vi "Continuous_Measurement_v4.vi"() -> ()   [LabVIEW 2014]
uses:
  <vilib>/Analysis/NI_AALBase.lvlib
panel:
  out "Redraw V-I graph?":bool
  in  "Reset Graphs?":bool
  out "File Startname":string
  in  "stop":bool
  out "I-t Graph":dbl[](graph)
  out "V-t Graph":dbl[](graph)
  out "V-I Graph":cluster{dbl[], dbl[]}(graph)
  in  "Meas. wait time (ms)":i32
  in  "Meas. to Avg":i32
  out "Voltage (V)":string
  in  "Current (uA)":dbl
  in  "Collect":bool
  in  "Outp. wait time (ms)":i32
  in  "2182A VISA":refnum<visa-resource-name>
  in  "Output Response":bool
  in  "Compliance (V)":dbl
  out "File Counter":i32
  out "Data Counter":i32
  in  "6221 VISA":refnum<visa-resource-name>
  in  "First Path":path
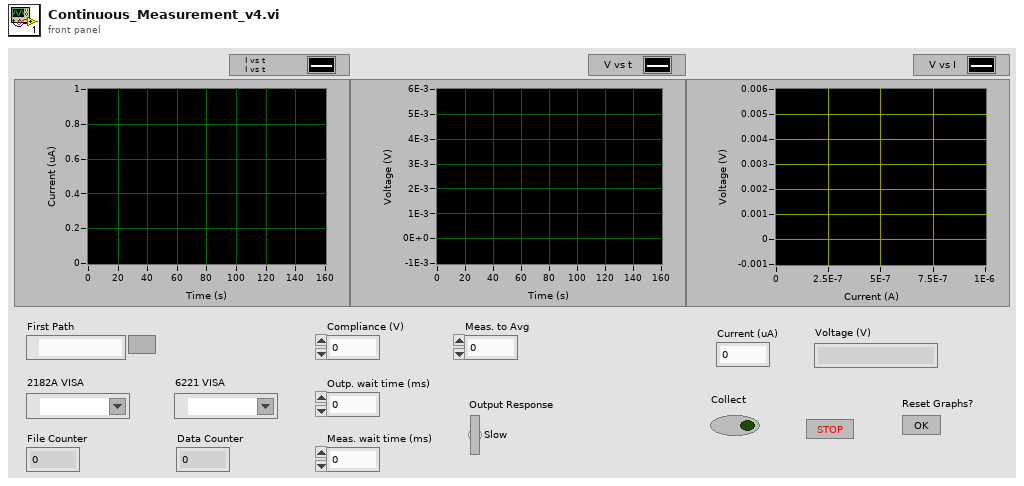
[diagram p1: front panel]
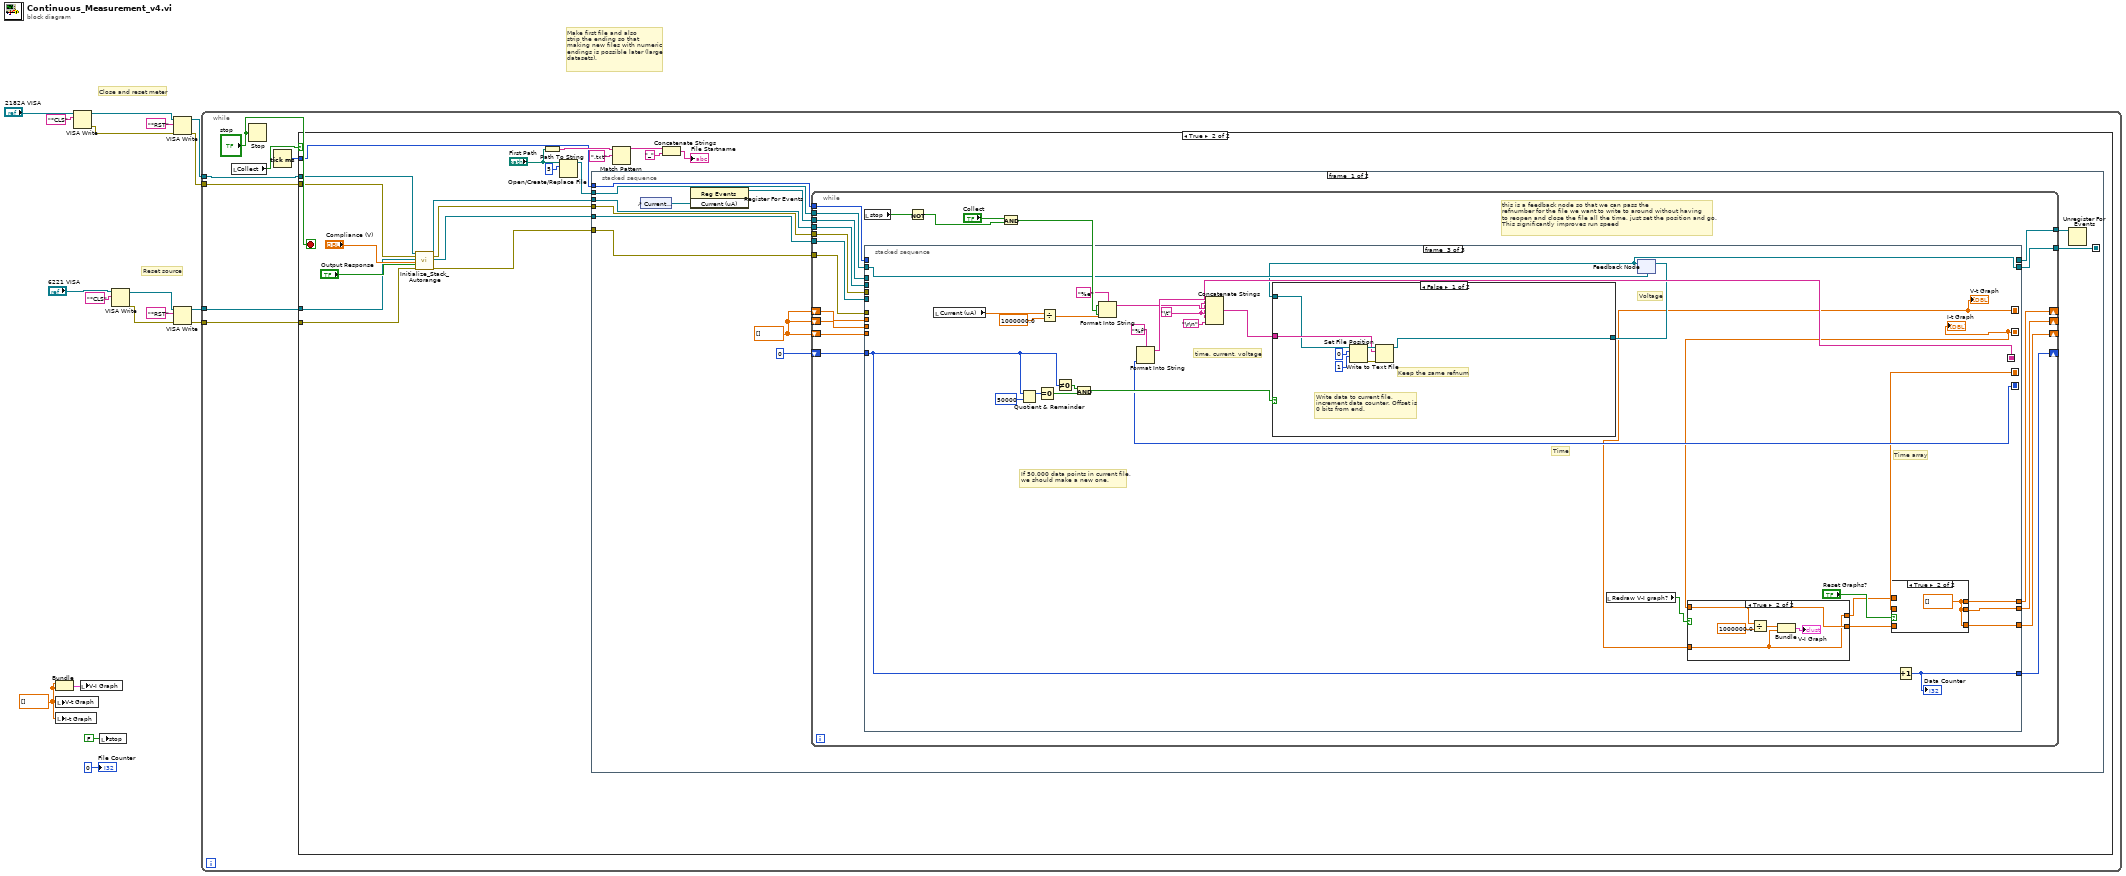
[diagram p0: block diagram]
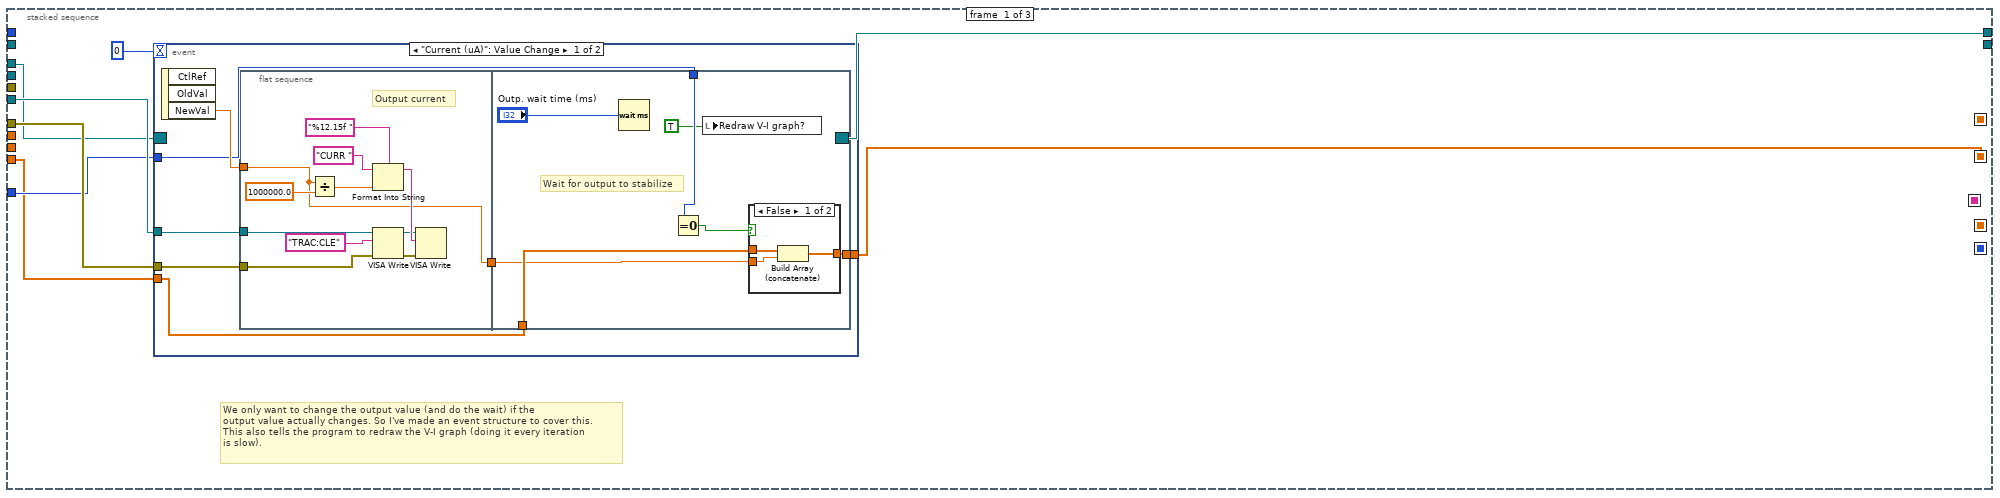
[diagram p3: hidden frame]
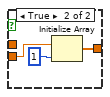
[diagram p4: hidden frame]
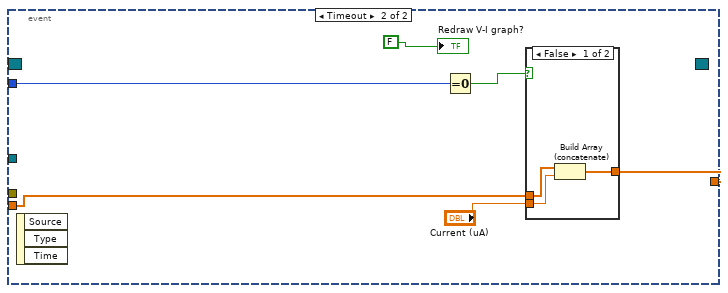
[diagram p5: hidden frame]
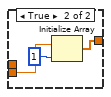
[diagram p6: hidden frame]
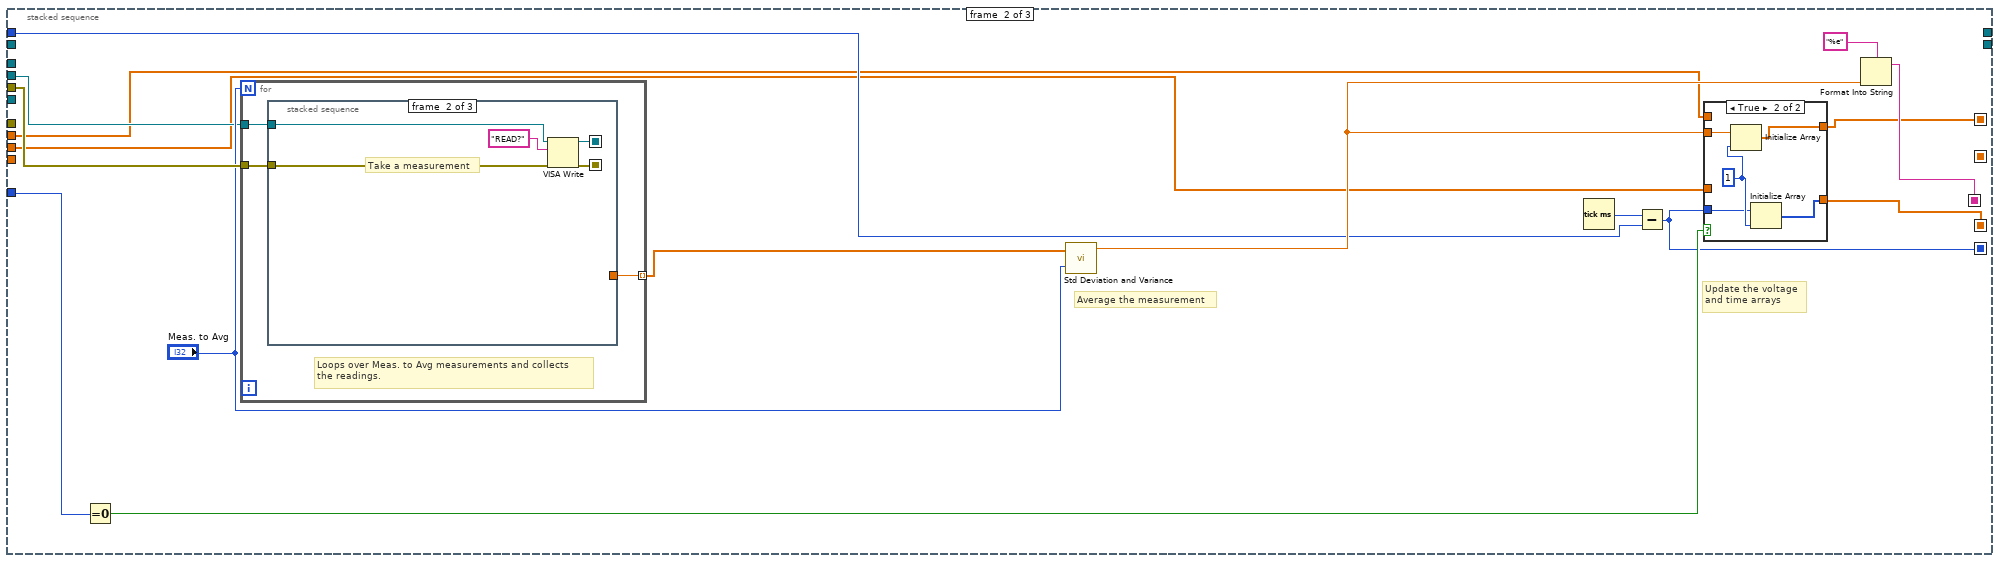
[diagram p7: hidden frame]
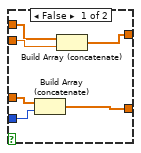
[diagram p8: hidden frame]
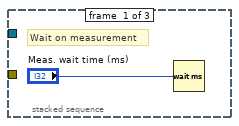
[diagram p9: hidden frame]
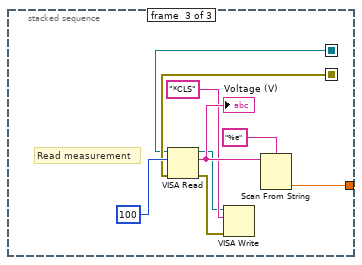
[diagram p10: hidden frame]
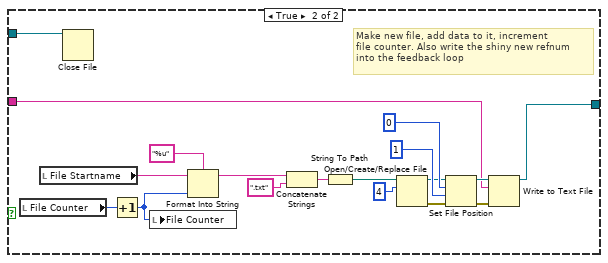
[diagram p13: hidden frame]
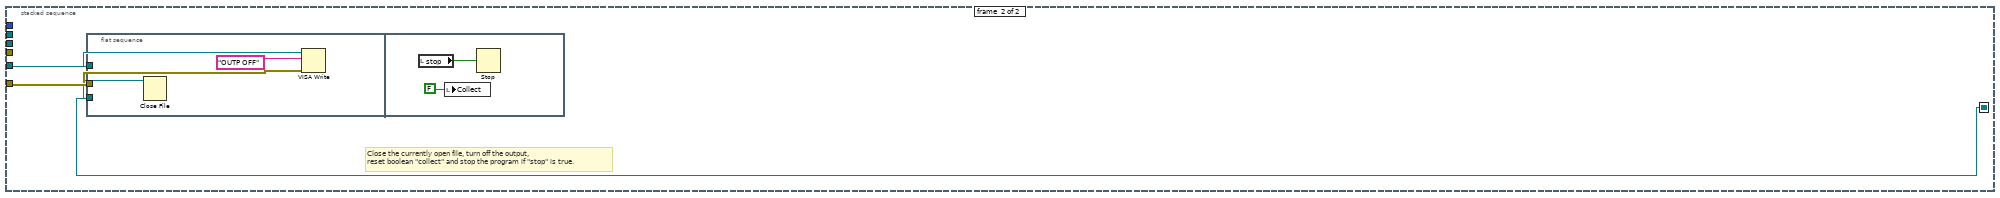
[diagram p14: hidden frame]
diagram:
  w2 = dbl[] []
  # "Make first file and also\nstrip the ending so that\nmaking new files with numeric\nendings is possible later (large\ndatasets)."
  # "Reset source"
  # "Close and reset meter"
  n1 = Bundle(w2, w2) -> (w1:cluster{dbl[], dbl[]})  [unwired: 1 in]
  n2 = local write "V-t Graph"(w2) -> ()
  n3 = local write "I-t Graph"(w2) -> ()
  n4 = VISA Write(VISA resource name="2182A VISA", write buffer="*CLS") -> (VISA resource name out=w11:refnum<visa-resource-name>, error out=w15:errorcluster)  [unwired: 1 in, 1 out]
  n5 = local write "V-I Graph"(w1) -> ()
  n6 = local write "stop"(FALSE) -> ()
  n7 = VISA Write(VISA resource name="6221 VISA", write buffer="*CLS") -> (VISA resource name out=w4:refnum<visa-resource-name>, error out=w5:errorcluster)  [unwired: 1 in, 1 out]
  n8 = VISA Write(VISA resource name=w11, write buffer="*RST", error in (no error)=w15) -> (VISA resource name out=w10:refnum<visa-resource-name>, error out=w9:errorcluster)  [unwired: 1 out]
  n9 = VISA Write(VISA resource name=w4, write buffer="*RST", error in (no error)=w5) -> (VISA resource name out=w7:refnum<visa-resource-name>, error out=w6:errorcluster)  [unwired: 1 out]
  n10 = while {
    tunnel: w10 -> [w24]
    tunnel: w9 -> [w23]
    tunnel: w7 -> [w22]
    tunnel: w6 -> [w21]
    stop <- "stop" stop-if-true
    n11 = local read "Collect"() -> (w25:bool)
    n12 = Stop(stop? (T)="stop") -> ()
    n13 = Tick Count (ms)() -> (millisecond timer value=w19:u32)
    n14 = case shown="True" w25 {
      tunnel: w23 -> [_ w30]
      tunnel: w24 -> [_ w31]
      tunnel: w22 -> [_ w32]
      tunnel: w21 -> [_ w33]
      tunnel: w19 -> [_ w36]
      frame False {
      }
      frame True {
        n15 = call "Initialize_Stack_Autorange.vi"("2182A VISA in"=w31, "21282A Error In"=w30, "6221 VISA in"=w32, "Compliance (V)"="Compliance (V)", "Output Response"="Output Response", "6221 Error In"=w33) -> ("2182A VISA out"=w29:refnum<visa-resource-name>, "2182A Error Out"=w28:errorcluster, "6221 VISA out"=w27:refnum<visa-resource-name>, "6221 Error Out"=w26:errorcluster)  [unwired: 10 in]
        n16 = Path To String(path="First Path") -> (string=w43:string)
        n17 = Open/Create/Replace File(file path (use dialog)="First Path", operation (0:open)=5) -> (refnum out=w40:refnum<file>)  [unwired: 4 in, 2 out]
        n18 = stacked-sequence {
          seq-local: [w51 _] -> [_ w242]
          tunnel: w26 -> [w56 w243]
          tunnel: w28 -> [w55 _]
          tunnel: w27 -> [w54 w244]
          tunnel: w29 -> [w53 _]
          tunnel: w40 -> [w52 _]
          tunnel: w36 -> [w48 _]
          frame #0 {
            w47 = dbl[] []
            n19 = control-ref of="Current (uA)"() -> (w50:refnum<vi>)
            n20 = register-events(w50) -> (reference out=w49:refnum<event-registration>)  [unwired: 2 in, 1 out]
            n21 = while {
              tunnel: w56 -> [w77]
              tunnel: w55 -> [w68]
              tunnel: w54 -> [w73]
              tunnel: w53 -> [w67]
              tunnel: w52 -> [w71]
              tunnel: [w70] -> w51
              tunnel: w49 -> [w69]
              tunnel: w48 -> [w66]
              shift-right: [w59] -> _
              shift-left: w47 -> [w60]
              shift-right: [w58] -> _
              shift-left: w47 -> [w62]
              shift-right: [w57] -> _
              shift-left: w47 -> [w65]
              shift-right: [w64] -> _
              shift-left: 0 -> [w63]
              tunnel: [w61] -> w45
              stop <- w74 continue-if-true
              # "this is a feedback node so that we can pass the\nrefnumber for the file we want to write to around without having\nto reopen and close the file all the time, just set the position and go. \nThis significantly improves run speed"
              n22 = local read "stop"() -> (w72:bool)
              n23 = stacked-sequence {
                seq-local: [_ w140 _] -> [_ _ w196]
                seq-local: [w80 _ _] -> [_ _ w176]
                seq-local: [_ w132 _] -> [_ _ w178]
                seq-local: [_ w131 _] -> [_ _ w183]
                seq-local: [_ w130 _] -> [_ _ w182]
                tunnel: w77 -> [w84 _ _]
                tunnel: w68 -> [_ w144 _]
                tunnel: w73 -> [w85 _ _]
                tunnel: w67 -> [_ w139 _]
                tunnel: w71 -> [_ _ w192]
                tunnel: [_ _ w190] -> w70
                tunnel: w69 -> [w83 _ _]
                tunnel: w66 -> [_ w136 _]
                tunnel: w65 -> [_ w133 _]
                tunnel: [_ _ w185] -> w64
                tunnel: w63 -> [w81 w135 w186]
                tunnel: w62 -> [w79 _ _]
                tunnel: [w78 _ _] -> w61
                tunnel: w60 -> [_ w129 _]
                tunnel: [_ _ w181] -> w59
                tunnel: [_ _ w180] -> w58
                tunnel: [_ _ w179] -> w57
                frame #0 {
                  # "We only want to change the output value (and do the wait) if the\noutput value actually changes. So I've made an event structure to cover this.\nThis also tells the program to redraw the V-I graph (doing it every iteration\nis slow)."
                  n24 = event shown="[0] \"Current (uA)\": Value Change" {
                    selector: w83 -> [_ _]
                    dyn-events: [_ _] -> w78
                    timeout: 0 -> [_ _]
                    tunnel: w85 -> [w91 _]
                    tunnel: w84 -> [w90 _]
                    tunnel: w81 -> [w89 w120]
                    tunnel: [w88 w119] -> w80
                    tunnel: w79 -> [w86 w118]
                    event "Current (uA)": Value Change {
                      n25 = event-data() -> ("NewVal"=w92:dbl)  [unwired: 1 in, 2 out]
                      n26 = flat-sequence {
                        tunnel: w92 -> [w93]
                        tunnel: w91 -> [w95]
                        tunnel: w90 -> [w94]
                        tunnel: [w93] -> w87
                        tunnel: w86 -> [w106]
                        tunnel: w89 -> [w109]
                        tunnel: [w107] -> w88
                        tunnel: w87 -> [w105]
                        frame #0 {
                          # "Output current"
                          n27 = Divide(x=w93, y=1000000.0) -> (x/y=w98:dbl)
                          n28 = Format Into String(format string="%12.15f ", initial string="CURR ", w98) -> (resulting string=w100:string)  [unwired: 1 in, 1 out]
                          n29 = VISA Write(VISA resource name=w95, write buffer="TRAC:CLE", error in (no error)=w94) -> (VISA resource name out=w97:refnum<visa-resource-name>, error out=w102:errorcluster)  [unwired: 1 out]
                          n30 = VISA Write(VISA resource name=w97, write buffer=w100, error in (no error)=w102) -> ()  [unwired: 3 out]
                        }
                        frame #1 {
                          # "Wait for output to stabilize"
                          n31 = Wait (ms)(milliseconds to wait="Outp. wait time (ms)") -> ()  [unwired: 1 out]
                          n32 = Equal To 0?(x=w109) -> (x = 0?=w108:bool)
                          n33 = local write "Redraw V-I graph?"(TRUE) -> ()
                          n34 = case shown="False" w108 {
                            tunnel: [w111 w115] -> w107
                            tunnel: w105 -> [w112 w114]
                            tunnel: w106 -> [w113 _]
                            frame False {
                              n35 = Build Array (concatenate)(w113, w112) -> (w111:dbl[])
                            }
                            frame True {
                              n36 = Initialize Array(w114, 1) -> (w115:dbl[])
                            }
                          }
                        }
                      }
                    }
                    event Timeout {
                      n37 = event-data() -> ()  [unwired: 1 in, 3 out]
                      n38 = Equal To 0?(x=w120) -> (x = 0?=w121:bool)
                      n39 = case shown="False" w121 {
                        tunnel: [w123 w127] -> w119
                        tunnel: "Current (uA)" -> [w124 w126]
                        tunnel: w118 -> [w125 _]
                        frame False {
                          n40 = Build Array (concatenate)(w125, w124) -> (w123:dbl[])
                        }
                        frame True {
                          n41 = Initialize Array(w126, 1) -> (w127:dbl[])
                        }
                      }
                      "Redraw V-I graph?" <- FALSE
                    }
                  }
                }
                frame #1 {
                  # "Update the voltage\nand time arrays"
                  # "Average the measurement"
                  n42 = Equal To 0?(x=w135) -> (x = 0?=w134:bool)
                  n43 = for {
                    N: "Meas. to Avg" -> [_]
                    tunnel: w144 -> [w158]
                    tunnel: [w157] -> w143 mode=indexing
                    tunnel: w139 -> [w156]
                    # "Loops over Meas. to Avg measurements and collects\nthe readings."
                    n44 = stacked-sequence {
                      seq-local: [_ w162 _] -> [_ _ w172]
                      seq-local: [_ w160 _] -> [_ _ w169]
                      tunnel: w158 -> [_ w163 _]
                      tunnel: [_ _ w170] -> w157
                      tunnel: w156 -> [_ w161 _]
                      frame #0 {
                        # "Wait on measurement"
                        n45 = Wait (ms)(milliseconds to wait="Meas. wait time (ms)") -> ()  [unwired: 1 out]
                      }
                      frame #1 {
                        # "Take a measurement"
                        n46 = VISA Write(VISA resource name=w161, write buffer="READ?", error in (no error)=w163) -> (VISA resource name out=w160:refnum<visa-resource-name>, error out=w162:errorcluster)  [unwired: 1 out]
                      }
                      frame #2 {
                        # "Read measurement"
                        n47 = VISA Read(VISA resource name=w169, byte count=100, error in (no error)=w172) -> (VISA resource name out=w166:refnum<visa-resource-name>, read buffer=w168:string, error out=w165:errorcluster)  [unwired: 1 out]
                        "Voltage (V)" <- w168
                        n48 = VISA Write(VISA resource name=w166, write buffer="*CLS", error in (no error)=w165) -> ()  [unwired: 3 out]
                        n49 = Scan From String(format string="%e", input string=w168) -> (output 1=w170:dbl)  [unwired: 3 in, 3 out]
                      }
                    }
                  }
                  n50 = call <vilib>:"Std Deviation and Variance.vi"("X"=w143, "Weighting (Sample)"="Meas. to Avg") -> ("mean"=w138:dbl)  [unwired: 2 out]
                  n51 = Tick Count (ms)() -> (millisecond timer value=w137:u32)
                  n52 = Subtract(x=w137, y=w136) -> (x-y=w131:u32)
                  n53 = case shown="True" w134 {
                    tunnel: w131 -> [w150 w154]
                    tunnel: w138 -> [w149 w153]
                    tunnel: [w148 w152] -> w132
                    tunnel: [w147 w151] -> w130
                    tunnel: w129 -> [w146 _]
                    tunnel: w133 -> [w145 _]
                    frame False {
                      n54 = Build Array (concatenate)(w145, w150) -> (w148:dbl[])
                      n55 = Build Array (concatenate)(w146, w149) -> (w147:dbl[])
                    }
                    frame True {
                      w155 = 1
                      n56 = Initialize Array(w153, w155) -> (w151:dbl[])
                      n57 = Initialize Array(w154, w155) -> (w152:u32[])
                    }
                  }
                  n58 = Format Into String(format string="%e", w138) -> (resulting string=w140:string)  [unwired: 2 in, 1 out]
                }
                frame #2 {
                  w201 = "\t"
                  # "Voltage"
                  # "Time array"
                  # "Time"
                  # "time, current, voltage"
                  # "If 50,000 data points in current file,\nwe should make a new one."
                  n59 = local read "Current (uA)"() -> (w184:dbl)
                  n60 = Quotient & Remainder(x=w186, y=50000) -> (x-y*floor(x/y)=w193:i32)  [unwired: 1 out]
                  n61 = Equal To 0?(x=w193) -> (x = 0?=w188:bool)
                  n62 = Divide(x=w184, y=1000000.0) -> (x/y=w195:dbl)
                  n63 = Not Equal To 0?(x=w186) -> (x != 0?=w187:bool)
                  n64 = And(x=w187, y=w188) -> (x .and. y?=w198:bool)
                  n65 = Format Into String(format string="%e", w195) -> (resulting string=w202:string)  [unwired: 2 in, 1 out]
                  n66 = Format Into String(format string="%f", w183) -> (resulting string=w204:string)  [unwired: 2 in, 1 out]
                  n67 = Concatenate Strings(w204, w201, w202, w201, w196, "\r\n") -> (w197:string)
                  n68 = local read "Redraw V-I graph?"() -> (w177:bool)
                  n69 = feedback #1(w192) -> (w190:refnum<file>)
                  n70 = case shown="False" w198 {
                    tunnel: w197 -> [w220 w231]
                    tunnel: [w218 w230] -> w191
                    tunnel: w190 -> [w217 w241]
                    frame False {
                      # "Keep the same refnum"
                      # "Write data to current file,\nincrement data counter. Offset is\n0 bits from end."
                      n71 = Set File Position(offset (in bytes) (0)=0, refnum=w217, from (0:start)=1) -> (refnum out=w221:refnum<file>, error out=w219:errorcluster)  [unwired: 1 in]
                      n72 = Write to Text File(file (use dialog)=w221, text=w220, error in=w219) -> (refnum out=w218:refnum<file>)  [unwired: 1 in, 2 out]
                    }
                    frame True {
                      # "Make new file, add data to it, increment\nfile counter. Also write the shiny new refnum\ninto the feedback loop"
                      n73 = local read "File Counter"() -> (w229:i32)
                      n74 = local read "File Startname"() -> (w224:string)
                      n75 = Close File(refnum=w241) -> ()  [unwired: 1 in, 2 out]
                      n76 = Increment(x=w229) -> (x+1=w225:i32)
                      n77 = local write "File Counter"(w225) -> ()
                      n78 = Format Into String(format string="%u", initial string=w224, w225) -> (resulting string=w240:string)  [unwired: 1 in, 1 out]
                      n79 = Concatenate Strings(w240, ".txt") -> (w236:string)
                      n80 = String To Path(string=w236) -> (path=w238:path)
                      n81 = Open/Create/Replace File(file path (use dialog)=w238, operation (0:open)=u16 4) -> (refnum out=w228:refnum<file>, error out=w227:errorcluster)  [unwired: 4 in, 1 out]
                      n82 = Set File Position(offset (in bytes) (0)=i64 0, refnum=w228, from (0:start)=u16 1, error in=w227) -> (refnum out=w234:refnum<file>, error out=w235:errorcluster)
                      n83 = Write to Text File(file (use dialog)=w234, text=w231, error in=w235) -> (refnum out=w230:refnum<file>)  [unwired: 1 in, 2 out]
                    }
                  }
                  n84 = feedback-in #1(w191) -> ()
                  n85 = case shown="True" w177 {
                    tunnel: w176 -> [w207 w209]
                    tunnel: w182 -> [w206 w208]
                    tunnel: [w207 w209] -> w175
                    tunnel: [w206 w208] -> w174
                    frame False {
                    }
                    frame True {
                      n86 = Divide(x=w209, y=1000000.0) -> (x/y=w211:dbl[])
                      n87 = Bundle(w211, w208) -> (→"V-I Graph":cluster{dbl[], dbl[]})  [unwired: 1 in]
                    }
                  }
                  n88 = case shown="True" "Reset Graphs?" {
                    tunnel: [w214 w216] -> w181
                    tunnel: [w215 w216] -> w180
                    tunnel: w175 -> [w215 _]
                    tunnel: w174 -> [w214 _]
                    tunnel: [w213 w216] -> w179
                    tunnel: w178 -> [w213 _]
                    frame False {
                    }
                    frame True {
                      w216 = dbl[] []
                    }
                  }
                  n89 = Increment(x=w186) -> (x+1=w185:i32)
                  "Data Counter" <- w185
                  "V-t Graph" <- w182
                  "I-t Graph" <- w176
                }
              }
              n90 = Not(x=w72) -> (.not. x?=w75:bool)
              n91 = And(x="Collect", y=w75) -> (x .and. y?=w74:bool)
            }
            n92 = Unregister For Events(event registration refnum=w45) -> ()  [unwired: 1 in, 1 out]
          }
          frame #1 {
            # "Close the currently open file, turn off the output,\nreset boolean \"collect\" and stop the program if \"stop\" is true."
            n93 = flat-sequence {
              tunnel: w244 -> [w247]
              tunnel: w243 -> [w246]
              tunnel: w242 -> [w245]
              frame #0 {
                n94 = Close File(refnum=w245) -> ()  [unwired: 1 in, 2 out]
                n95 = VISA Write(VISA resource name=w247, write buffer="OUTP OFF", error in (no error)=w246) -> ()  [unwired: 3 out]
              }
              frame #1 {
                n96 = local read "stop"() -> (w250:bool)
                n97 = local write "Collect"(FALSE) -> ()
                n98 = Stop(stop? (T)=w250) -> ()
              }
            }
          }
        }
        n99 = Match Pattern(string=w43, regular expression=".txt") -> (before substring=w39:string)  [unwired: 1 in, 3 out]
        n100 = Concatenate Strings(w39, "_") -> (→"File Startname":string)
      }
    }
  }
  "File Counter" <- 0
